vi "Open File Do.vi"(8 "error in (no error)":errorcluster, 10 "New File Path":path, 11 "TDMS File Writer in":refnum<class "File Writer_TDMS.lvclass">) -> (0 "error out":errorcluster, 1 "Success?":bool, 3 "TDMS File Writer out":refnum<class "File Writer_TDMS.lvclass">)   [LabVIEW 2020, in "File Writer_TDMS.lvlib" / "File Writer_TDMS.lvclass"]
doc: "Open or create a TDMS file."
uses:
  File Writer_TDMS.lvclass
  File Writer_TDMS.lvclass/File Writer_TDMS.ctl
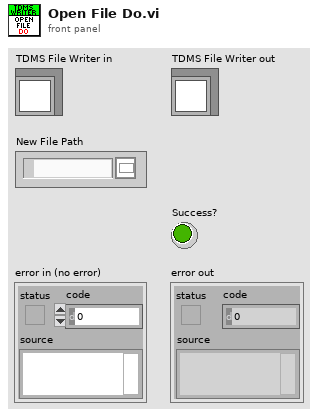
[diagram p1: front panel]
types:
  T1 = enum16{"big-endian, network order", "native, host order", "little-endian"}
  T2 = enum16{"open", "open or create", "create or replace", "create", "open (read-only)"}
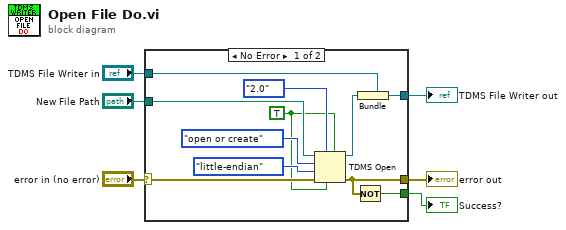
[diagram p0: block diagram]
diagram:
  n1 = case shown="No Error" "error in (no error)" {
    selector: "error in (no error)" -> [w14 w18]
    tunnel: "New File Path" -> [w17 _]
    tunnel: [w8 w18] -> w5
    tunnel: "TDMS File Writer in" -> [w11 w19]
    tunnel: [w9 w19] -> w3
    tunnel: [w7 _] -> w2
    frame No Error {
      w12 = TRUE ("disable buffering? (T)")
      n2 = TDMS Open(5:w12, 6:w12, 7:enum16{"1.0", "2.0"}."2.0" ("file format version (2.0)"), 8:w14, 9:T1."little-endian" ("byte order (2:little-endian)"), 10:T2."open or create" ("operation (0:open)"), 11:w17) -> (0:w8:errorcluster, 3:w10:refnum<k34>)
      n3 = Not(x=w8) -> (.not. x?=w7:bool)
      n4 = Bundle(cluster=w11, w10) -> (w9:refnum<class "File Writer_TDMS.lvclass">)
    }
    frame Error {
    }
  }
  "error out" <- w5
  "TDMS File Writer out" <- w3
  "Success?" <- w2
